vi "Extract and display key can statisctics.vi"(9 "Supply current output":dbl, 10 "Supply voltage output":dbl, 11 "Signal map in":map{string, dbl}(c390)) -> (3 "Key statistics":T1)   [LabVIEW 2024]
uses:
  Key CAN statistics.ctl
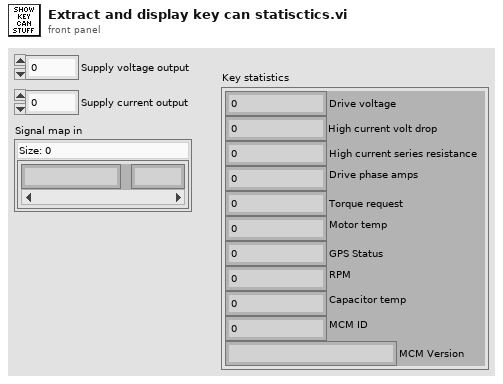
[diagram p1: front panel]
types:
  T1 = typedef "Key CAN statistics.ctl" = cluster{"Drive voltage ":dbl, "High current volt drop":dbl, "High current series resistance":dbl, "Drive phase amps":dbl, "Torque request":dbl, "Motor temp":dbl, "GPS Status":dbl, "RPM":dbl, "Capacitor temp":dbl, "MCM ID":dbl, "MCM Version":string}
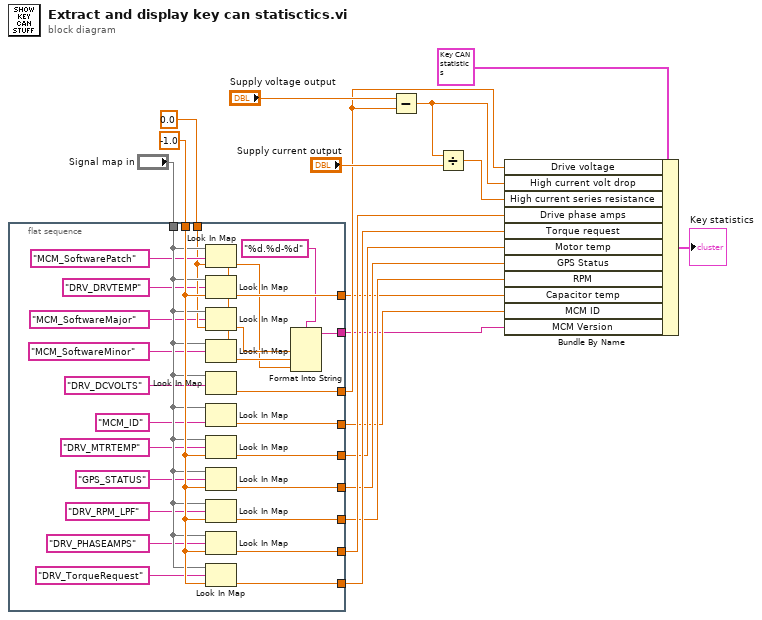
[diagram p0: block diagram]
diagram:
  n1 = flat-sequence {
    tunnel: "Signal map in" -> [w44]
    tunnel: -1.0 -> [w45]
    tunnel: 0.0 ("default value") -> [w33]
    tunnel: [w43] -> w9
    tunnel: [w42] -> w8
    tunnel: [w41] -> w7
    tunnel: [w40] -> w6
    tunnel: [w39] -> w5
    tunnel: [w38] -> w4
    tunnel: [w37] -> w3
    tunnel: [w36] -> w2
    tunnel: [w20] -> w1
    frame #0 {
      n2 = Look In Map(map=w44, key="MCM_SoftwarePatch", default value=w33) -> (value=w21:dbl)  [unwired: 1 out]
      n3 = Look In Map(map=w44, key="DRV_DRVTEMP", default value=w45) -> (value=w37:dbl)  [unwired: 1 out]
      n4 = Look In Map(map=w44, key="MCM_SoftwareMajor", default value=w33) -> (value=w23:dbl)  [unwired: 1 out]
      n5 = Look In Map(map=w44, key="MCM_SoftwareMinor", default value=w33) -> (value=w22:dbl)  [unwired: 1 out]
      n6 = Look In Map(map=w44, key="DRV_DCVOLTS") -> (value=w43:dbl)  [unwired: 1 in, 1 out]
      n7 = Look In Map(map=w44, key="MCM_ID") -> (value=w36:dbl)  [unwired: 1 in, 1 out]
      n8 = Look In Map(map=w44, key="DRV_MTRTEMP", default value=w45) -> (value=w40:dbl)  [unwired: 1 out]
      n9 = Look In Map(map=w44, key="GPS_STATUS", default value=w45) -> (value=w39:dbl)  [unwired: 1 out]
      n10 = Look In Map(map=w44, key="DRV_RPM_LPF", default value=w45) -> (value=w38:dbl)  [unwired: 1 out]
      n11 = Look In Map(map=w44, key="DRV_PHASEAMPS", default value=w45) -> (value=w42:dbl)  [unwired: 1 out]
      n12 = Look In Map(map=w44, key="DRV_TorqueRequest", default value=w45) -> (value=w41:dbl)  [unwired: 1 out]
      n13 = Format Into String(format string="%d.%d-%d", w23, w22, w21) -> (resulting string=w20:string)  [unwired: 2 in, 1 out]
    }
  }
  n14 = Subtract(x="Supply voltage output", y=w9) -> (x-y=w13:dbl)
  n15 = Divide(x=w13, y="Supply current output") -> (x/y=w14:dbl)
  n16 = Bundle By Name(cluster=T1 {"Drive voltage "=0.0, "High current volt drop"=0.0, "High current series resistance"=0.0, "Drive phase amps"=0.0, "Torque request"=0.0, "Motor temp"=0.0, "GPS Status"=0.0, "RPM"=0.0, "Capacitor temp"=0.0, "MCM ID"=0.0, "MCM Version"=""} ("Key statistics"), "Drive voltage"=w9, "High current volt drop"=w13, "High current series resistance"=w14, "Drive phase amps"=w8, "Torque request"=w7, "Motor temp"=w6, "GPS Status"=w5, "RPM"=w4, "Capacitor temp"=w3, "MCM ID"=w2, "MCM Version"=w1) -> (→"Key statistics":T1)
